vi "WindowVI.vi"() -> ()   [LabVIEW 2017]
panel:
  in  "hidden one":dbl
  in  "Numeric 4":dbl
  in  "Numeric 3":dbl
  in  "Numeric 2":dbl
  in  "Numeric":dbl
  # "This is a hidden item"
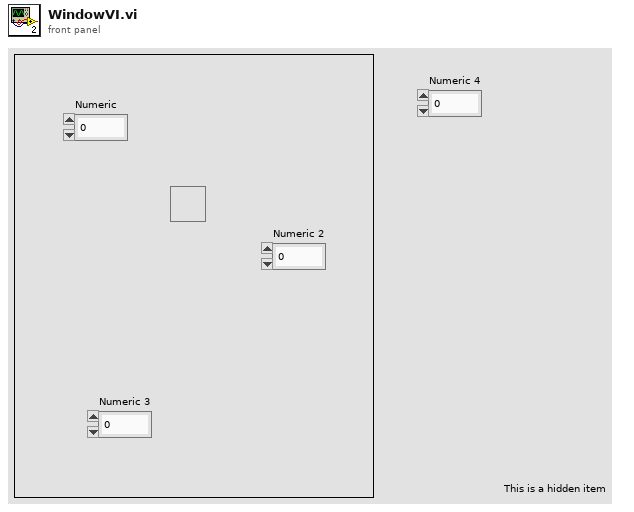
[diagram p1: front panel]
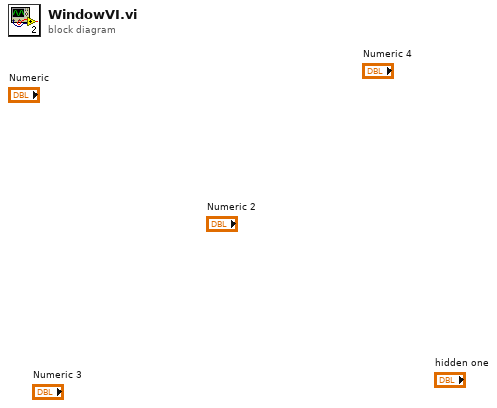
[diagram p0: block diagram]
diagram:
